vi "Move Motor Y.vi"(10 "Move Y":dbl, 11 "Move X":dbl) -> ()   [LabVIEW 2014]
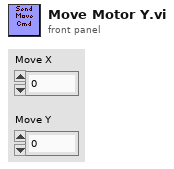
[diagram p1: front panel]
types:
  T1 = enum16{"Default", "Set Statuses", "Set Parameters", "Save Parameter"}
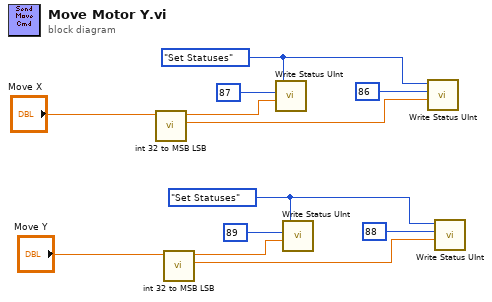
[diagram p0: block diagram]
diagram:
  w4 = T1."Set Statuses" ("Command")
  w10 = T1."Set Statuses" ("Command")
  n1 = call "int 32 to MSB LSB.vi"("Signed 32 Bit Int"="Move X") -> ("LSB NUM"=w8:dbl, "MSB NUM"=w9:dbl)  [unwired: 9 in]
  n2 = call "int 32 to MSB LSB.vi"("Signed 32 Bit Int"="Move Y") -> ("LSB NUM"=w2:dbl, "MSB NUM"=w3:dbl)  [unwired: 9 in]
  n3 = call "Write Status UInt.vi"("Status Value"=w9, "Status Number"=u16 87 ("Status Value"), "Command"=w10) -> ()  [unwired: 4 in, 1 out]
  n4 = call "Write Status UInt.vi"("Status Value"=w3, "Status Number"=u16 89 ("Status Value"), "Command"=w4) -> ()  [unwired: 4 in, 1 out]
  n5 = call "Write Status UInt.vi"("Status Value"=w8, "Status Number"=u16 86 ("Status Value"), "Command"=w10) -> ()  [unwired: 4 in, 1 out]
  n6 = call "Write Status UInt.vi"("Status Value"=w2, "Status Number"=u16 88 ("Status Value"), "Command"=w4) -> ()  [unwired: 4 in, 1 out]
